vi "Flatten Pixmap - GIF__ogtk.vi"(8 "StartColorIndex":i32, 9 "ExistingColorTable":u32[](array[numeric]), 11 "PixelTable":u32[][](array[colorbox])) -> (0 "EndColorIndex":i32, 3 "image data":T1)   [LabVIEW 2018]
uses:
  <vilib>/picture/picture.llb/imagedata.ctl
panel:
  # "Util.Pic.PixelTableToImage(single).vi\n\nConverts a single 2D Pixel-table an LV \"image data\" cluster.\n\nPlease visit http://www.OpenG.org to learn about the\nOpen Source LabVIEW software movement.\n\nNOTICE -- YOU MUST LEAVE THIS NOTICE IN PLACE.  PER THE TERMS OF THE LICENSE BELOW, YOU MAY SUBLICENSE THIS SOFTWARE \nIN ANY WAY THAT DOES NOT CONFLICT WITH THIS LICENSE.\n\n### BSD License (http://www.opensource.org/licenses/bsd-license.php) Begin ###\n \nCopyright (c) 2007, Bill Clench <bclench@yahoo.com>\n\nAll rights reserved.\n\nRedistribution and use in source and binary forms, with or without modification, are permitted provided that the following conditions are met:\n\n    * Redistributions of source code must retain the above copyright notice, this list of conditions and the following disclaimer.\n    * Redistributions in binary form must reproduce the above copyright notice, this list of conditions and the following disclaimer in the \n       documentation and/or other materials provided with the distribution.\n    * Neither the name of SciWare, James Kring, Inc., nor the names of its contributors may be used to endorse or promote products derived \n       from this software without specific prior written permission.\n\nTHIS SOFTWARE IS PROVIDED BY THE COPYRIGHT HOLDERS AND CONTRIBUTORS \"AS IS\" AND ANY EXPRESS OR IMPLIED WARRANTIES, \nINCLUDING, BUT NOT LIMITED TO, THE IMPLIED WARRANTIES OF MERCHANTABILITY AND FITNESS FOR A PARTICULAR PURPOSE ARE \nDISCLAIMED. IN NO EVENT SHALL THE COPYRIGHT OWNER OR CONTRIBUTORS BE LIABLE FOR ANY DIRECT, INDIRECT, INCIDENTAL,\n SPECIAL, EXEMPLARY, OR CONSEQUENTIAL DAMAGES (INCLUDING, BUT NOT LIMITED TO, PROCUREMENT OF SUBSTITUTE GOODS OR \nSERVICES; LOSS OF USE, DATA, OR PROFITS; OR BUSINESS INTERRUPTION) HOWEVER CAUSED AND ON ANY THEORY OF LIABILITY, \nWHETHER IN CONTRACT, STRICT LIABILITY, OR TORT (INCLUDING NEGLIGENCE OR OTHERWISE) ARISING IN ANY WAY OUT OF THE USE \nOF THIS SOFTWARE, EVEN IF ADVISED OF THE POSSIBILITY OF SUCH DAMAGE.\n\n### BSD License End ###"
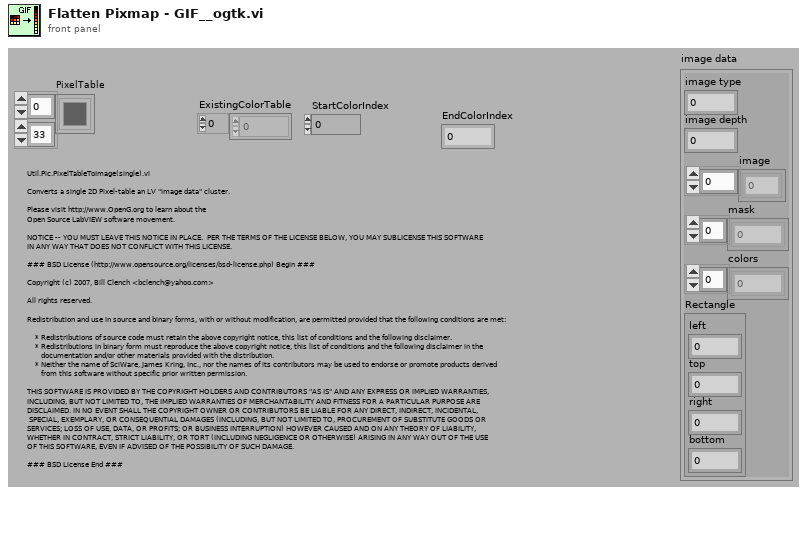
[diagram p1: front panel]
types:
  T1 = typedef "imagedata.ctl" = cluster{"image type":i32, "image depth":i32, "image":u8[], "mask":u8[], "colors":u32[], "Rectangle":cluster{"left":i16, "top":i16, "right":i16, "bottom":i16}}
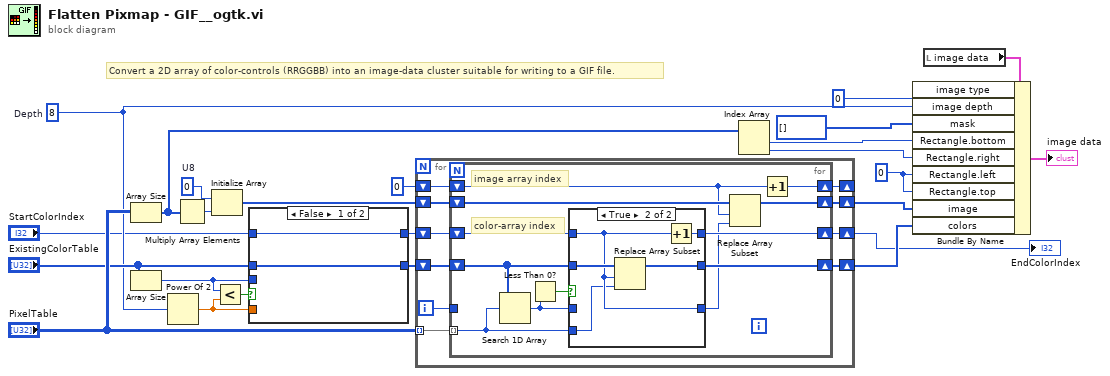
[diagram p0: block diagram]
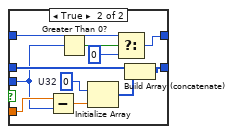
[diagram p2: hidden frame]
diagram:
  w7 = 8  # Depth
  w9 = i16 0 ("Rectangle.left")
  w24 = u8 0  # U8
  # "Convert a 2D array of color-controls (RRGGBB) into an image-data cluster suitable for writing to a GIF file."
  n1 = Array Size(array="PixelTable") -> (size(s)=w17:i32[])
  n2 = Array Size(array="ExistingColorTable") -> (size(s)=w4:i32)
  n3 = Power Of 2(x=w7) -> (2^x=w16:dbl)
  n4 = Multiply Array Elements(1:w17) -> (0:w23:i32)
  n5 = Initialize Array(w24, w23) -> (w22:u8[])
  n6 = Less?(x=w4, y=w16) -> (x < y?=w15:bool)
  n7 = case shown="False" w15 {
    tunnel: [w26 w34] -> w6
    tunnel: w16 -> [_ w32]
    tunnel: "ExistingColorTable" -> [w26 w37]
    tunnel: w4 -> [_ w28]
    tunnel: "StartColorIndex" -> [w25 w29]
    tunnel: [w25 w27] -> w2
    frame False {
    }
    frame True {
      w35 = u32 0  # U32
      n8 = Subtract(x=w32, y=w28) -> (x-y=w36:dbl)
      n9 = Greater Than 0?(x=w28) -> (x > 0?=w31:bool)
      n10 = Initialize Array(w35, w36) -> (w33:u32[])
      n11 = Select(t=w29, s=w31, f=0) -> (s? t:f=w27:i32)
      n12 = Build Array (concatenate)(w37, w33) -> (w34:u32[])
    }
  }
  n13 = for {
    shift-right: [w46] -> w5
    shift-left: w6 -> [w39]
    tunnel: "PixelTable" -> [w47] mode=indexing
    shift-right: [w44] -> w1
    shift-left: w2 -> [w45]
    shift-right: [w42] -> w13
    shift-left: w22 -> [w43]
    shift-right: [w40] -> _
    shift-left: 0 -> [w41]
    i -> [w38]
    n14 = for {
      tunnel: w47 -> [w48] mode=indexing
      shift-right: [w57] -> w46
      shift-left: w39 -> [w58]
      shift-right: [w54] -> w44
      shift-left: w45 -> [w55]
      shift-right: [w53] -> w42
      shift-left: w43 -> [w52]
      shift-right: [w51] -> w40
      shift-left: w41 -> [w50]
      tunnel: w38 -> [_]
      # "color-array index"
      # "image array index"
      n15 = Search 1D Array(1D array=w58, element=w48) -> (index of element=w56:i32)  [unwired: 1 in]
      n16 = Less Than 0?(x=w56) -> (x < 0?=w59:bool)
      n17 = case shown="True" w59 {
        tunnel: w58 -> [w62 w67]
        tunnel: w48 -> [_ w63]
        tunnel: [w62 w66] -> w57
        tunnel: w56 -> [w60 _]
        tunnel: w55 -> [w61 w64]
        tunnel: [w61 w65] -> w54
        tunnel: [w60 w64] -> w49
        frame False {
        }
        frame True {
          n18 = Replace Array Subset(array=w67, new element=w63, index=w64) -> (w66:u32[])
          n19 = Increment(x=w64) -> (x+1=w65:i32)
        }
      }
      n20 = Replace Array Subset(array=w52, new element=w49, index=w50) -> (w53:u8[])
      n21 = Increment(x=w50) -> (x+1=w51:i32)
    }
  }
  "EndColorIndex" <- w1
  n22 = Index Array(array=w17) -> (element #1=w11:i32, element #2=w21:i32)  [unwired: 2 in]
  n23 = local read "image data"() -> (w19:T1)
  n24 = Bundle By Name(cluster=w19, "image type"=0, "image depth"=w7, "mask"=u8[] [] ("initialized array"), "Rectangle.bottom"=w11, "Rectangle.right"=w21, "Rectangle.left"=w9, "Rectangle.top"=w9, "image"=w13, "colors"=w5) -> (→"image data":T1)
